vi "Charger_Move Error Source to Status.vi"(0 "error in":errorcluster, 4 "Status Refnum":T1) -> (7 "error out":errorcluster)   [LabVIEW 2020]
uses:
  Charger_Status Refnum.ctl
  Drivers/Charger Test Set/Charger_Input Control.ctl
panel:
  out "status string":string
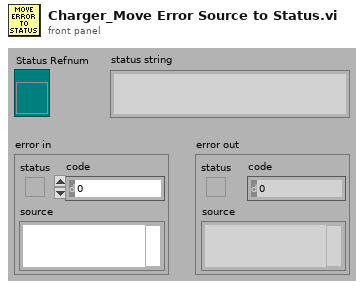
[diagram p1: front panel]
types:
  T1 = typedef "Charger_Status Refnum.ctl" = refnum<vi>
  T2 = typedef "Charger_Input Control.ctl" = cluster{"address":refnum<visa-resource-name>, "position":i32, "setpoint":dbl}
  T3 = cluster{"MICS ID":u32, "VBAT":dbl, "ChargingState":string, "VBAT Slide":dbl, "Status":string, "TemperatureLevel":dbl, "IPG_ReceivedLevel":dbl, "VBAT Target":dbl, "Charger Setpoint":dbl, "Index":i32, "Ready":bool, "Charger Inputs":T2, "MICS Inputs":cluster{"address":refnum<visa-resource-name>, "chan":u16, "ID":u32}}
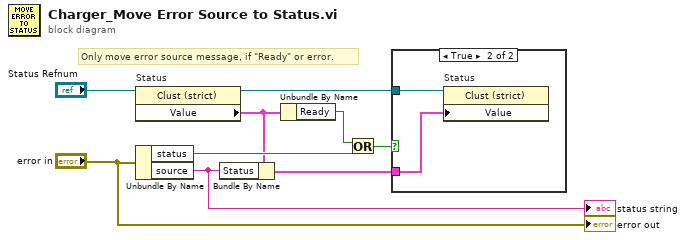
[diagram p0: block diagram]
diagram:
  # "Only move error source message, if \"Ready\" or error."
  n1 = property on="Status" class="Clust (strict)"(reference="Status Refnum") -> (reference out=w9:T1, "Value"=w2:T3)  [unwired: 1 in, 1 out]
  n2 = Unbundle By Name ("error in")("error in") -> ("status"=w5:bool, "source"=w4:string)
  "status string" <- w4
  n3 = Bundle By Name(cluster=w2, "Status"=w4) -> (w3:T3)
  n4 = Unbundle By Name(w2) -> ("Ready"=w6:bool)
  n5 = Or(x=w6, y=w5) -> (x .or. y?=w1:bool)
  n6 = case shown="True" w1 {
    tunnel: w9 -> [_ w11]
    tunnel: w3 -> [_ w10]
    frame False {
    }
    frame True {
      n7 = property on="Status" class="Clust (strict)"(reference=w11, "Value"=w10) -> ()  [unwired: 1 in, 2 out]
    }
  }
  "error out" <- "error in"
